vi "Not a Window Refnum.vi"() -> (0 "Not a Window Refnum":T1)   [LabVIEW 2023, in "WINUTIL.lvlib"]
uses:
  WINUTIL.lvlib
  Window Refnum.ctl
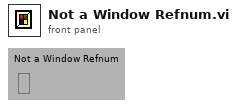
[diagram p1: front panel]
types:
  T1 = typedef "WINUTIL.lvlib/Window Refnum.ctl" = refnum<k1>
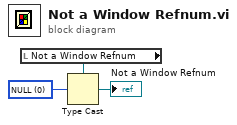
[diagram p0: block diagram]
diagram:
  w3 = u32 0 items=["NULL"]
  n1 = local read "Not a Window Refnum"() -> (w2:T1)
  n2 = Type Cast(type=w2, x=w3) -> (*(type *) &x=→"Not a Window Refnum":T1)
